vi "shift page wheel.vi"(7 "read write":string(combo), 9 "wheel page in":string[][][](array[string]), 10 "current run list in":string[][](array[string])) -> (1 "wheel page out":string[][][](array[string]), 2 "current run list out":string[][](array[string]))   [LabVIEW 2016]
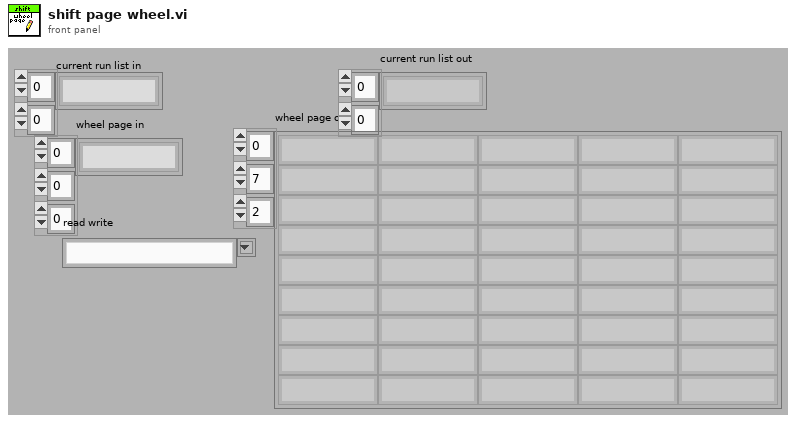
[diagram p1: front panel]
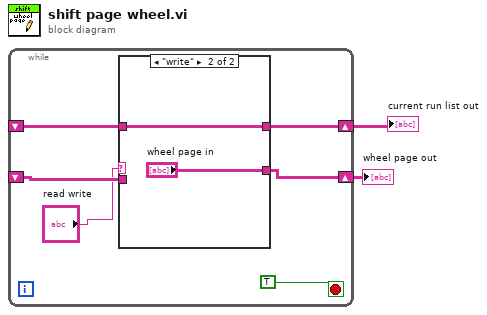
[diagram p0: block diagram]
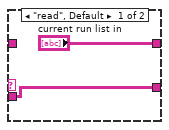
[diagram p2: hidden frame]
diagram:
  n1 = while {
    shift-right: [w7] -> w2
    shift-left: _ -> [w6]
    shift-right: [w4] -> w1
    shift-left: _ -> [w3]
    stop <- TRUE ("stop") stop-if-true
    n2 = case shown="\"write\"" "read write" {
      tunnel: [w10 "wheel page in"] -> w7
      tunnel: w6 -> [w10 _]
      tunnel: ["current run list in" w11] -> w4
      tunnel: w3 -> [_ w11]
      frame "read", Default {
      }
      frame "write" {
      }
    }
  }
  "wheel page out" <- w2
  "current run list out" <- w1
